vi "Process Signals with a Filter Bank.vi"() -> ()   [LabVIEW 2023]
doc: "This example demonstrates how to use the Filter Bank Processing VIs to decompose and reconstruct signals.\n\nComplete the following steps to use this VI:\n1) Specify an <b>Input Signal</b>.\n2) Run this VI.\n3) Observe the <b>Signal</b>. The output signal is a delayed version of the input signal. \n4) Observe the <b>Reconstruction Error</b>. The reconstruction error is small."
uses:
  <vilib>/addons/Digital Filter Design/Process.llb/DFD Integer Delay (Array).vi
  <vilib>/addons/Digital Filter Design/FilterBank.llb/Process/DFD 2-Band Filter Bank Decomposition (Array).vi
  <vilib>/addons/Digital Filter Design/FilterBank.llb/Process/DFD 2-Band Filter Bank Reconstruction (Array).vi
  <vilib>/Analysis/NI_AALBase.lvlib
  <vilib>/addons/Digital Filter Design/NI_DigFilter_FilterBank.lvlib
  <vilib>/addons/Digital Filter Design/NI_DigFilterLicensed.lvlib
panel:
  in  "Input Signal":enum16{"White Noise", "Sine", "Chirp"}(ring)=enum."Sine"
  out "Reconstruction Error":dbl[](graph)
  out "Signal":dbl[][](graph)
  # "Select Help>>Show Context Help and move the cursor over the VI icon for more information."
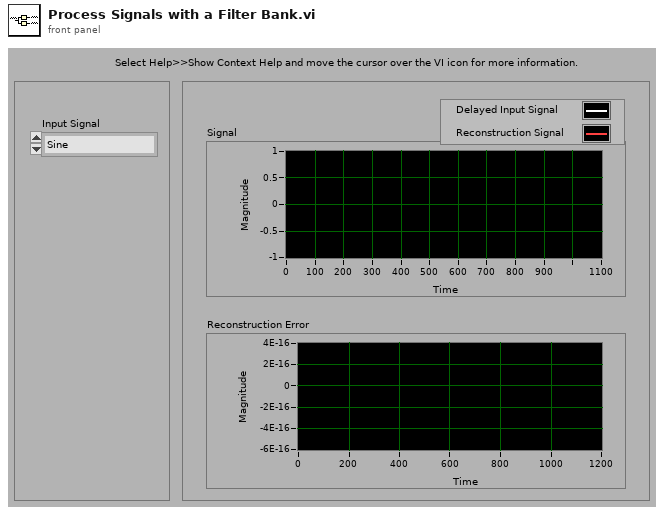
[diagram p1: front panel]
types:
  T1 = typedef "NI_DigFilter_FilterBank.lvlib/DFD Filter Bank Obj.ctl" = cluster{"mFBank_AnalysisFilters":T2[], "mFBank_SynthesisFilters":T2[], "mFBank_#Bands":i32, "mFBank_ProcMethod":T7, "mFBank_Coeffs":dbl[], "mFBank_Gain":dbl, "mFBank_Delay":i32, "mFBank_Type":T8}
  T2 = typedef "NI_DigFilterLicensed.lvlib/DFD Multirate Filter Obj.ctl" = cluster{"mMRate_Structure":enum16{"CIC", "FIR", "IIR", "Lattice"}, "mMRate_Mode":T3, "mMRate_Factor":i32, "mMRate_FIRParams":cluster{"mMRate_FIR_H":dbl[], "mMRate_FIR_IsNyquist?":bool, "mMRate_FIR_IsSymmetric?":bool}, "mMRate_CICParams":cluster{"mMRate_CIC_#Stage":i32, "mMRate_CIC_Lag":i32, "mMRate_CIC_Type":enum16{"Lowpass", "Highpass"}}, "mMRate_Order":i32, "mMRate_Version":string, "mMRate_Comments":string, "mMRate_RationalFactor":cluster{"mMRate_L":i32, "mMRate_M":i32}, "mMRate_Fs":dbl, "mMRate_Quantized?":bool, "mMRate_QFilterGain":dbl, "mMRate_CoefWl":i16, "mMRate_Scaling":cluster{"mMRate_ScaleByPowerOf2?":bool, "mMRate_ScaleType":T4}, "mMRate_InputWl":i16, "mMRate_OutputWl":i16, "mMRate_OutputMode":T5, "mMRate_MultMode":T6, "mMRate_BitPruning":bool, "mMRate_GainWl":i16, "mMRate_OutputFwl":i16, "mMRate_SumIwl":i16, "mMRate_InputIwl ":i16, "mMRate_SumWl":i16, "mMRate_CoefIwl":i16}
  T3 = typedef "NI_DigFilterLicensed.lvlib/DFD Multirate Mode.ctl" = i16
  T4 = typedef "NI_DigFilterLicensed.lvlib/DFD Coef Norm Type.ctl" = enum16{"No Norm", "Time Domain 1-Norm", "Time Domain 2-Norm", "Time Domain Inf-Norm"}
  T5 = typedef "NI_DigFilterLicensed.lvlib/DFD Round-off Mode.ctl" = enum16{"Nearest", "Truncation"}
  T6 = typedef "NI_DigFilterLicensed.lvlib/DFD FXP MRate Multiply Mode.ctl" = enum16{"Truncated", "Full"}
  T7 = typedef "NI_DigFilter_FilterBank.lvlib/DFD Filter Bank Processing Method.ctl" = enum16{"General", "2-Band QMF Lattice", "Cosine-Modulated"}
  T8 = typedef "NI_DigFilter_FilterBank.lvlib/DFD Filter Bank Type.ctl" = u16
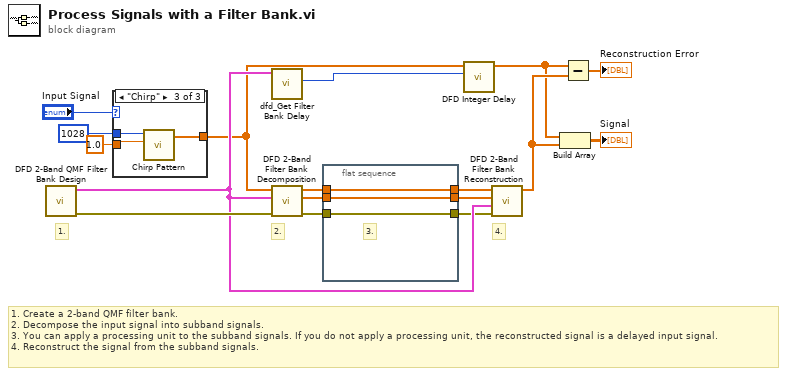
[diagram p0: block diagram]
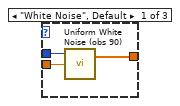
[diagram p2: hidden frame]
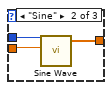
[diagram p3: hidden frame]
diagram:
  # "4."
  # "2."
  # "1."
  # "1. Create a 2-band QMF filter bank.\n2. Decompose the input signal into subband signals.\n3. You can apply a processing unit to the subband signals. If you do not apply a processing unit, the reconstructed signal is a delayed input signal.\n4. Reconstruct the signal from the subband signals."
  n1 = call <vilib>:"DFD 2-Band QMF Filter Bank Design.vi"() -> ("error out"=w17:errorcluster, "filter bank out"=w16:T1)  [unwired: 9 in, 1 out]
  n2 = case shown="\"Chirp\"" "Input Signal" {
    tunnel: [w20 w23 w26] -> w10
    tunnel: 1028 -> [w19 w22 w25]
    tunnel: 1.0 -> [w18 w21 w24]
    frame "White Noise", Default {
      n3 = call <vilib>:"Uniform White Noise (obs 90).vi"("amplitude"=w18, "samples"=w19) -> ("uniform white noise"=w20:dbl[])  [unwired: 1 in, 1 out]
    }
    frame "Sine" {
      n4 = call <vilib>:"Sine Wave.vi"("samples"=w22, "amplitude"=w21) -> ("sine wave"=w23:dbl[])  [unwired: 3 in, 2 out]
    }
    frame "Chirp" {
      n5 = call <vilib>:"Chirp Pattern.vi"("amplitude"=w24, "samples"=w25) -> ("Chirp Pattern"=w26:dbl[])  [unwired: 2 in, 1 out]
    }
  }
  n6 = call <vilib>:"dfd_Get Filter Bank Delay.vi"("bank in"=w16) -> ("delay"=w12:i32)  [unwired: 8 in, 2 out]
  n7 = call-poly <vilib>:"DFD 2-Band Filter Bank Decomposition.vi"("error in (no error)"=w17, "filter bank in"=w16, "signal in"=w10) -> ("error out"=w3:errorcluster, "highpass band"=w5:dbl[], "lowpass band"=w7:dbl[])  [unwired: 6 in]
  n8 = flat-sequence {
    tunnel: w7 -> [w29]
    tunnel: [w29] -> w6
    tunnel: [w28] -> w4
    tunnel: w5 -> [w28]
    tunnel: w3 -> [w27]
    tunnel: [w27] -> w2
    frame #0 {
      # "3."
    }
  }
  n9 = call-poly <vilib>:"DFD Integer Delay.vi"("delay"=w12, "signal in"=w10) -> ("signal out"=w1:dbl[])  [unwired: 8 in, 1 out]
  n10 = call-poly <vilib>:"DFD 2-Band Filter Bank Reconstruction.vi"("error in (no error)"=w2, "filter bank in"=w16, "highpass band"=w4, "lowpass band"=w6) -> ("signal out"=w9:dbl[])  [unwired: 6 in, 1 out]
  n11 = Build Array(w1, w9) -> (→"Signal":dbl[][])
  n12 = Subtract(x=w1, y=w9) -> (x-y=→"Reconstruction Error":dbl[])
